vi "temperature change (v2021).vi"() -> ()   [LabVIEW 2021]
panel:
  in  "?":bool
  in  "?":bool
  in  "NodeMCU IP Address":string
  # "Start"
  # "Stop"
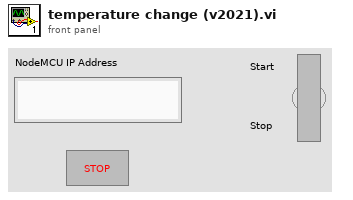
[diagram p1: front panel]
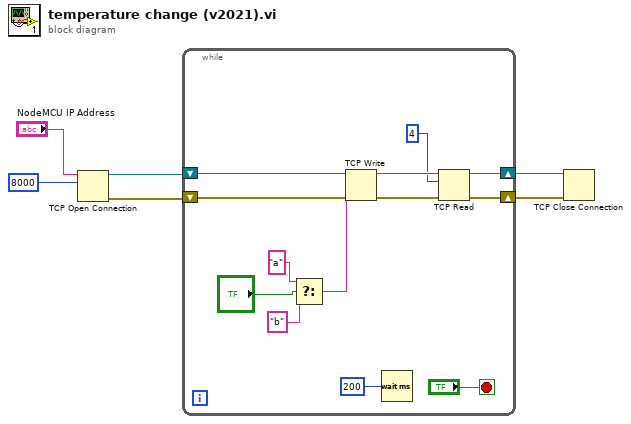
[diagram p0: block diagram]
diagram:
  n1 = TCP Open Connection(address="NodeMCU IP Address", remote port or service name=u16 8000) -> (connection ID=w4:refnum<k5>, error out=w3:errorcluster)  [unwired: 3 in]
  n2 = while {
    shift-right: [w15] -> w2
    shift-left: w4 -> [w19]
    shift-right: [w14] -> w1
    shift-left: w3 -> [w18]
    stop <- "?" stop-if-true
    n3 = Select(t="a", s="?", f="b") -> (s? t:f=w7:string)
    n4 = TCP Write(connection ID=w19, data in=w7, error in (no error)=w18) -> (connection ID out=w17:refnum<k5>, error out=w16:errorcluster)  [unwired: 1 in, 1 out]
    n5 = Wait (ms)(milliseconds to wait=u32 200) -> ()  [unwired: 1 out]
    n6 = TCP Read(connection ID=w17, bytes to read=4, error in (no error)=w16) -> (connection ID out=w15:refnum<k5>, error out=w14:errorcluster)  [unwired: 2 in, 1 out]
  }
  n7 = TCP Close Connection(connection ID=w2, error in (no error)=w1) -> ()  [unwired: 1 in, 2 out]
